vi "dfd_Halfband Filter Design with Order Param Estimation.vi"(7 "method":u16(ring)=3 items=["Kaiser Window", "Dolph-Chebyshev Window", "Equi-Ripple", "Positive Equi-Ripple"], 8 "error in (no error)":errorcluster, 10 "roll off":dbl=0.24 format="%.2f", 11 "order":i32) -> (0 "error out":errorcluster, 1 "band parameters":T1[](array[typedef]), 2 "window param":dbl=3.3953210522614574 format="%.2f", 3 "order out":i32=26)   [LabVIEW 2017, in "NI_DigFilter_Process.lvlib"]
uses:
  <vilib>/addons/Digital Filter Design/NI_DigFilter_Process.lvlib
  <vilib>/addons/Digital Filter Design/_Objects.llb/DFD Adv Band Spec.ctl
  <vilib>/addons/Digital Filter Design/_Misc.llb/dfd_Error Handlers (Single).vi
  <vilib>/addons/Digital Filter Design/NI_DigFilterLicensed.lvlib
panel:
  # "freq"
  # "amplitude"
  # "weight"
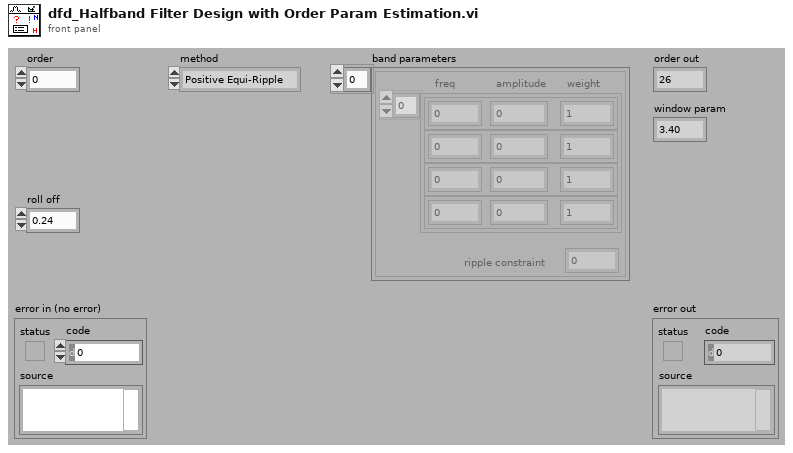
[diagram p1: front panel]
types:
  T1 = typedef "NI_DigFilterLicensed.lvlib/DFD Adv Band Spec.ctl" = cluster{"band specification":cluster{"freq":dbl, "amplitude":dbl, "weight":dbl}[], "ripple constraint":dbl}
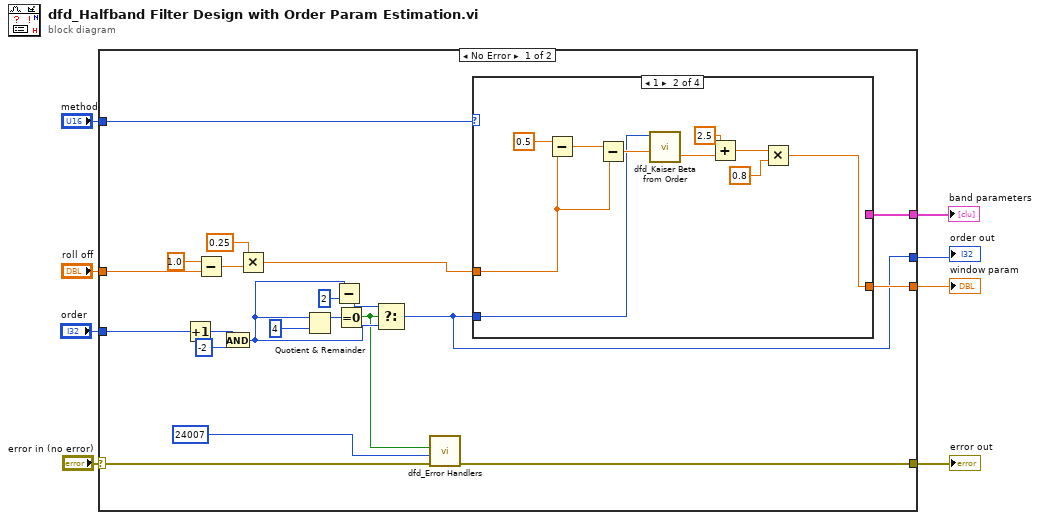
[diagram p0: block diagram]
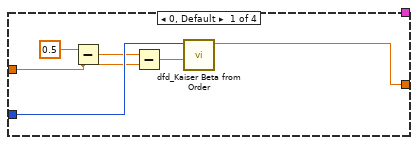
[diagram p2: hidden frame]
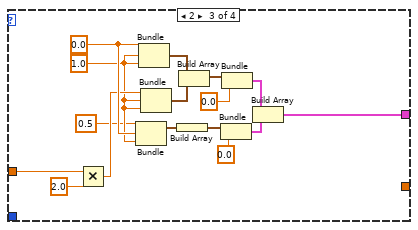
[diagram p3: hidden frame]
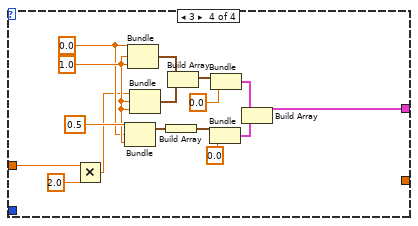
[diagram p4: hidden frame]
diagram:
  n1 = case shown="No Error" "error in (no error)" {
    selector: "error in (no error)" -> [w17 w78]
    tunnel: "method" -> [w29 _]
    tunnel: [w18 _] -> w7
    tunnel: [w16 w78] -> w6
    tunnel: "order" -> [w20 _]
    tunnel: "roll off" -> [w12 _]
    tunnel: [w28 _] -> w3
    tunnel: [w27 _] -> w1
    frame No Error {
      n2 = Increment(x=w20) -> (x+1=w23:i32)
      n3 = Subtract(x=1.0, y=w12) -> (x-y=w11:dbl)
      n4 = And(x=w23, y=-2) -> (x .and. y?=w21:i32)
      n5 = Multiply(x=0.25, y=w11) -> (x*y=w9:dbl)
      n6 = Quotient & Remainder(x=w21, y=4 ("x")) -> (x-y*floor(x/y)=w24:i32)  [unwired: 1 out]
      n7 = Subtract(x=w21, y=2) -> (x-y=w26:i32)
      n8 = Equal To 0?(x=w24) -> (x = 0?=w15:bool)
      n9 = Select(t=w26, s=w15, f=w21) -> (s? t:f=w18:i32)
      n10 = call-poly <vilib>:"dfd_Error Handlers.vi"("error in (no error)"=w17, "error code"=24007 ("WRN_ZERO_COEF_REMOVED"), "condition failed?"=w15) -> ("error out"=w16:errorcluster)  [unwired: 8 out]
      n11 = case shown="1" w29 {
        tunnel: w18 -> [w35 w44 _ _]
        tunnel: [_ _ w54 w62] -> w28
        tunnel: w9 -> [w33 w43 w60 w64]
        tunnel: [w30 w37 _ _] -> w27
        frame 0, Default {
          n12 = Subtract(x=0.5, y=w33) -> (x-y=w32:dbl)
          n13 = Subtract(x=w32, y=w33) -> (x-y=w34:dbl)
          n14 = call <vilib>:"dfd_Kaiser Beta from Order.vi"("delta f [Hz]"=w34, "order"=w35) -> ("beta"=w30:dbl)  [unwired: 9 out]
        }
        frame 1 {
          n15 = Subtract(x=0.5, y=w43) -> (x-y=w42:dbl)
          n16 = Subtract(x=w42, y=w43) -> (x-y=w45:dbl)
          n17 = call <vilib>:"dfd_Kaiser Beta from Order.vi"("delta f [Hz]"=w45, "order"=w44) -> ("r [dB]"=w40:dbl)  [unwired: 9 out]
          n18 = Add(x=2.5, y=w40) -> (x+y=w39:dbl)
          n19 = Multiply(x=w39, y=0.8) -> (x*y=w37:dbl)
        }
        frame 2 {
          w48 = 1.0
          w56 = 0.0
          n20 = Multiply(x=w60, y=2.0) -> (x*y=w49:dbl)
          n21 = Bundle(0.5, w56, w48) -> (w50:cluster{dbl, dbl, dbl})  [unwired: 1 out]
          n22 = Bundle(w56, w48, w48) -> (w59:cluster{dbl, dbl, dbl})  [unwired: 1 out]
          n23 = Bundle(w49, w48, w48) -> (w46:cluster{dbl, dbl, dbl})  [unwired: 1 out]
          n24 = Build Array(w50) -> (w51:cluster{dbl, dbl, dbl}[])
          n25 = Build Array(w59, w46) -> (w58:cluster{dbl, dbl, dbl}[])
          n26 = Bundle(w51, 0.0) -> (w52:cluster{cluster{dbl, dbl, dbl}[], dbl})  [unwired: 1 out]
          n27 = Bundle(w58, 0.0) -> (w55:cluster{cluster{dbl, dbl, dbl}[], dbl})  [unwired: 1 out]
          n28 = Build Array(w55, w52) -> (w54:cluster{cluster{dbl, dbl, dbl}[], dbl}[])
        }
        frame 3 {
          w74 = 1.0
          w68 = 0.0
          n29 = Multiply(x=w64, y=2.0) -> (x*y=w63:dbl)
          n30 = Bundle(0.5, w68, w74) -> (w73:cluster{dbl, dbl, dbl})  [unwired: 1 out]
          n31 = Bundle(w68, w74, w74) -> (w65:cluster{dbl, dbl, dbl})  [unwired: 1 out]
          n32 = Bundle(w63, w74, w74) -> (w76:cluster{dbl, dbl, dbl})  [unwired: 1 out]
          n33 = Build Array(w73) -> (w72:cluster{dbl, dbl, dbl}[])
          n34 = Build Array(w65, w76) -> (w66:cluster{dbl, dbl, dbl}[])
          n35 = Bundle(w72, 0.0) -> (w71:cluster{cluster{dbl, dbl, dbl}[], dbl})  [unwired: 1 out]
          n36 = Bundle(w66, 0.0) -> (w69:cluster{cluster{dbl, dbl, dbl}[], dbl})  [unwired: 1 out]
          n37 = Build Array(w69, w71) -> (w62:cluster{cluster{dbl, dbl, dbl}[], dbl}[])
        }
      }
    }
    frame Error {
    }
  }
  "order out" <- w7
  "window param" <- w1
  "error out" <- w6
  "band parameters" <- w3
